vi "CruiseControl.vi"(6 "reinitialize? (F)":bool, 7 "PID gains Velocity control":T1={"proportional gain (Kc)"=1.0, "integral time (Ti, min)"=0.01, "derivative time (Td, min)"=0.0} {"derivative time (Td, min)" step=0.01 format="%.3f"; "integral time (Ti, min)" format="%.3f"; "proportional gain (Kc)" step=0.05 format="%.3f"}, 8 "DistanceError":dbl, 9 "EstimatedVelocity":dbl, 10 "VelocityReference":dbl, 11 "K":dbl) -> (1 "VelocityReference to Controller":dbl, 2 "Velocity Voltage without limit (not sent to RIO)":dbl, 3 "Velocity Voltage":dbl)   [LabVIEW 2013]
uses:
  <vilib>/addons/control/pid/pid.llb/PID (DBL).vi
  <vilib>/imath/engines/lvmath2/RunTimeEngine/ErrorHandling/NIMS_Finalize Error.vi
  <vilib>/imath/engines/lvmath2/RunTimeEngine/Managers/WorkSpace/UID Generator.vi
  <vilib>/imath/engines/lvmath2/RunTimeEngine/RunTimeType/NIMS_RunTimeType_From StrictType (excl LVString).vi
  <instcachedir>/0/NIMS_RunTimeType_From StrictType (excl LVString)_4DEE718D6EB74582AA20236969C084FC.lvgen/NIMS_RunTimeType_From StrictType (excl LVString)_4DEE718D6EB74582AA20236969C084FC_000.vi
  <vilib>/imath/engines/lvmath2/RunTimeEngine/LocalVariableDefStatement/MC_LocalVariableDefStatement_Display.vi
  <vilib>/imath/engines/lvmath2/RunTimeEngine/Managers/SymbolTable/Clear UID.vi
  <vilib>/imath/engines/lvmath2/RunTimeEngine/NodeEndStatement/NIMS_NodeEndStatement_Output.vi
  <instcachedir>/0/NIMS_NodeEndStatement_Output_53EC0D466D134D7ABD903AC30B43404B.lvgen/NIMS_NodeEndStatement_Output_53EC0D466D134D7ABD903AC30B43404B_001.vi
  <vilib>/addons/control/pid/NI_PID_pid.lvlib
  <vilib>/imath/engines/lvmath2/RunTimeEngine/Managers/SymbolTable/NIMS_WorkSpace.lvlib
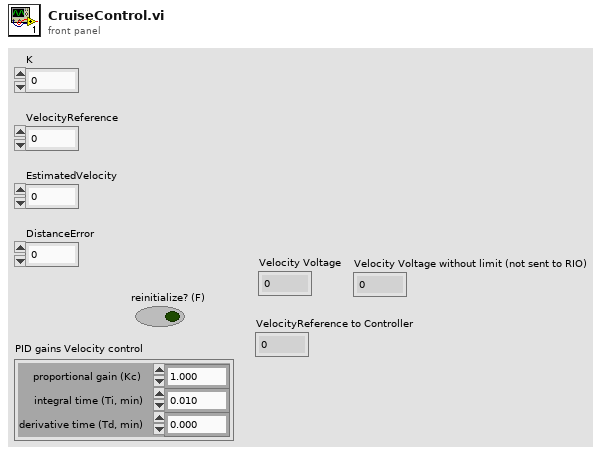
[diagram p1: front panel]
types:
  T1 = cluster{"proportional gain (Kc)":dbl, "integral time (Ti, min)":dbl, "derivative time (Td, min)":dbl}
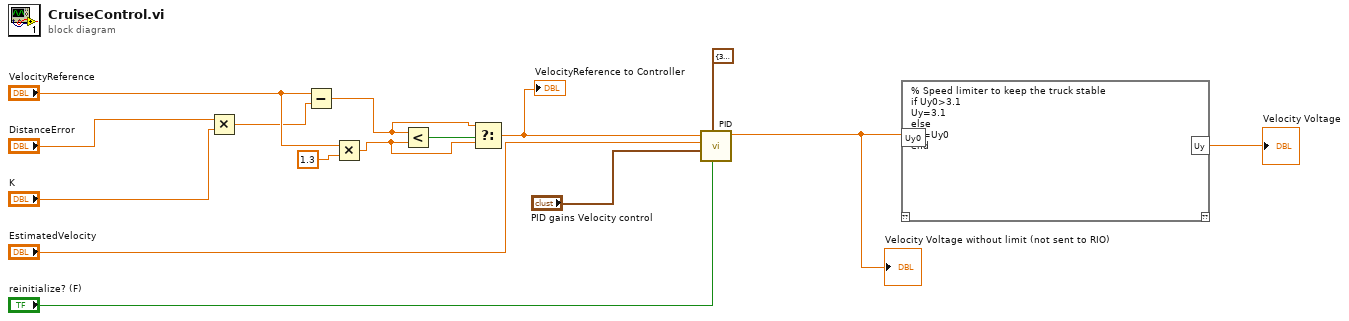
[diagram p0: block diagram]
diagram:
  n1 = Multiply(x="DistanceError", y="K") -> (x*y=w5:dbl)
  n2 = Subtract(x="VelocityReference", y=w5) -> (x-y=w2:dbl)
  n3 = Multiply(x="VelocityReference", y=1.3) -> (x*y=w1:dbl)
  n4 = Less?(x=w2, y=w1) -> (x < y?=w3:bool)
  n5 = Select(t=w2, s=w3, f=w1) -> (s? t:f=w11:dbl)
  "VelocityReference to Controller" <- w11
  n6 = call-poly <vilib>:"PID.vi"("reinitialize? (F)"="reinitialize? (F)", "output range"=cluster{"output high":dbl, "output low":dbl} {"output high"=3.6, "output low"=2.2}, "PID gains"="PID gains Velocity control", "process variable"="EstimatedVelocity", "setpoint"=w11) -> ("output"=w12:dbl)  [unwired: 5 in, 1 out]
  "Velocity Voltage without limit (not sent to RIO)" <- w12
  n7 = mathscript code="% Speed limiter to keep the truck stable\nif Uy0>3.1\nUy=3.1\nelse\nUy=Uy0\nend"("Uy0"=w12) -> ("Uy"=→"Velocity Voltage":dbl)  [unwired: 1 in, 1 out]
